vi "Write json to reg param one.vi"(8 "error in (no error)":errorcluster, 9 "RegsDescriptions":string[][](array[string]), 10 "JSON Data In":string, 11 "RegsParam in":dbl[][](array[numeric])) -> (0 "error out":errorcluster, 3 "RegsParam out":dbl[][](array[numeric]))   [LabVIEW 2019, in "control.lvlib"]
uses:
  control.lvlib
  bronkhorst/bronkhorstColumns.ctl
  <vilib>/JDP Science/JSONtext/Find Multiple Items.vi
  <vilib>/JDP Science/JSONtext/String Subset.vi
  <vilib>/JDP Science/JSONtext/support/Strip Quotes and Unescape.vi
  <vilib>/JDP Science/JSONtext/support/Unescape JSON string.vi
  <vilib>/JDP Science/JSONtext/Parsing/Parse Full Path or Item Name.vi
  <vilib>/JDP Science/JSONtext/Offset/Find Item Locations by Path.vi
  <vilib>/JDP Science/JSONtext/Get Array Elements.vi
  Userlib.lvlib
  bronkhorst/bronkhorst_reg.lvclass
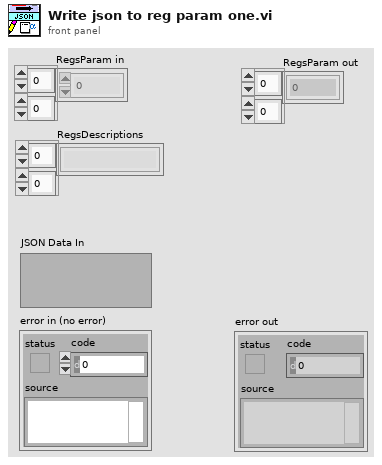
[diagram p1: front panel]
types:
  T1 = typedef "bronkhorst_reg.lvclass/bronkhorstColumns.ctl" = enum16{"instrument_range_max", "auto_value", "alr_value", "output_k", "output_set_time", "group", "process_units", "process_gas", "fcode", "fcode_full", "shortname"}
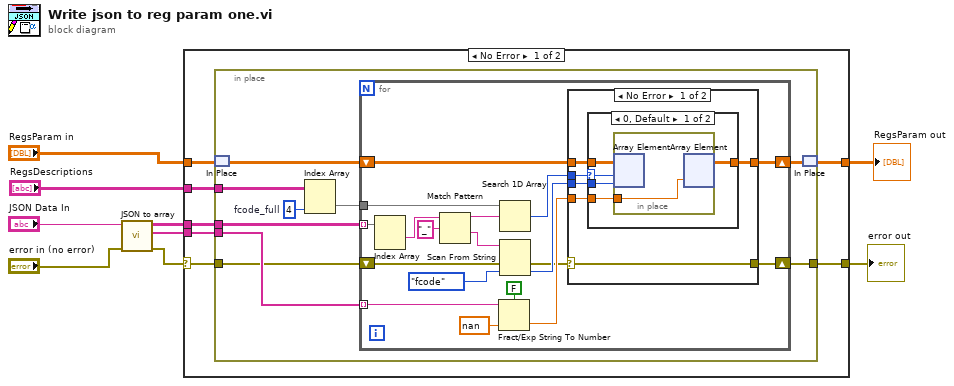
[diagram p0: block diagram]
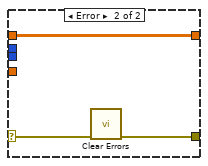
[diagram p3: hidden frame]
diagram:
  n1 = call "JSON to array.vi"("error in (no error)"="error in (no error)", "JSON Data In"="JSON Data In") -> ("error out"=w7:errorcluster, "values"=w4:string[], "names"=w5:string[][])  [unwired: 7 in]
  n2 = case shown="No Error" w7 {
    selector: w7 -> [w14 w61]
    tunnel: [w10 w61] -> w9
    tunnel: "RegsParam in" -> [w12 w60]
    tunnel: w4 -> [w15 _]
    tunnel: w5 -> [w16 _]
    tunnel: "RegsDescriptions" -> [w13 _]
    tunnel: [w11 w60] -> w1
    frame No Error {
      n3 = in-place {
        in-place-border: w14 -> [w20]
        in-place-border: w16 -> [w22]
        in-place-border: [w23] -> w10
        in-place-border: w15 -> [w21]
        in-place-border: w13 -> [w19]
        w25 = 4  # fcode_full
        n4 = in-place-match #1(w12) -> (w18:dbl[][])
        n5 = Index Array(array=w19, index (col)=w25) -> (element=w24:string[])  [unwired: 1 in]
        n6 = for {
          tunnel: w24 -> [w41]
          tunnel: w21 -> [w37] mode=indexing
          shift-right: [w38] -> w23
          shift-left: w20 -> [w34]
          shift-right: [w42] -> w17
          shift-left: w18 -> [w43]
          tunnel: w22 -> [w32] mode=indexing
          n7 = Index Array(array=w32) -> (element #1=w28:string)  [unwired: 2 in, 1 out]
          n8 = Match Pattern(string=w28, regular expression="_") -> (before substring=w26:string, after substring=w27:string)  [unwired: 1 in, 2 out]
          n9 = Fract/Exp String To Number(use system decimal point (T)=FALSE, string=w37, default (0 dbl)=nan ("default (0 DBL)")) -> (number=w36:dbl)  [unwired: 1 in, 1 out]
          n10 = Search 1D Array(1D array=w41, element=w26) -> (index of element=w40:i32)  [unwired: 1 in]
          n11 = Scan From String(input string=w27, error in=w34, default 1=bronkhorstColumns."fcode" ("ParamColumns")) -> (error out=w33:errorcluster, output 1=w39:T1)  [unwired: 2 in, 2 out]
          n12 = case shown="No Error" w33 {
            selector: w33 -> [w44 w58]
            tunnel: w43 -> [w49 w59]
            tunnel: [w48 w59] -> w42
            tunnel: w39 -> [w47 _]
            tunnel: w36 -> [w46 _]
            tunnel: w40 -> [w45 _]
            tunnel: [w44 w57] -> w38
            frame No Error {
              n13 = case shown="0, Default" w45 {
                selector: w45 -> [w50 _]
                tunnel: w49 -> [w54 w56]
                tunnel: [w53 w56] -> w48
                tunnel: w47 -> [w52 _]
                tunnel: w46 -> [w51 _]
                frame 0, Default {
                  n14 = in-place {
                    in-place-border: w51 -> [w55]
                    n15 = in-place-array #2(w54, w50, w52) -> ()  [unwired: 1 out]
                    n16 = in-place-array #2(w55) -> (w53:dbl[][])  [unwired: 2 out]
                  }
                }
                frame -1 {
                }
              }
            }
            frame Error {
              n17 = call <vilib>:"Clear Errors.vi"("error in (no error)"=w58) -> ("error out"=w57:errorcluster)  [unwired: 5 in, 1 out]
            }
          }
        }
        n18 = in-place-match #1(w17) -> (w11:dbl[][])
      }
    }
    frame Error {
    }
  }
  "error out" <- w9
  "RegsParam out" <- w1
